vi "Get Measruement Informations.vi"(11 "Measurement properties":T1={"Measurement ID"=enum."1", "Description"="3 phase, 3 ADC, 1 PJVS", "Switching matrix M"=[], "Signal frequency  (Hz)"=50.0, "Signal amplitudes (V)"=[], "PRs"=1, "PRe"=50, "MRs"=0, "MRe"=0, "Set PJVS frequency (Hz)"=50.0, "PJVS reference voltages (1 period, V)"=[], "Requiested PJVS steps"=10} {"PJVS reference voltages (1 period, V)" format="%.9g"}) -> (3 "Measurement properties out":T1={"Measurement ID"=enum."1", "Description"="3 phase, 3 ADC, 1 PJVS", "Switching matrix M"=[], "Signal frequency  (Hz)"=50.0, "Signal amplitudes (V)"=[], "PRs"=1, "PRe"=50, "MRs"=0, "MRe"=0, "Set PJVS frequency (Hz)"=50.0, "PJVS reference voltages (1 period, V)"=[], "Requiested PJVS steps"=10} {"PJVS reference voltages (1 period, V)" format="%.9g"})   [LabVIEW 2020]
uses:
  Type definitions/Measuement properties.ctl
  Type definitions/Measurement ID.ctl
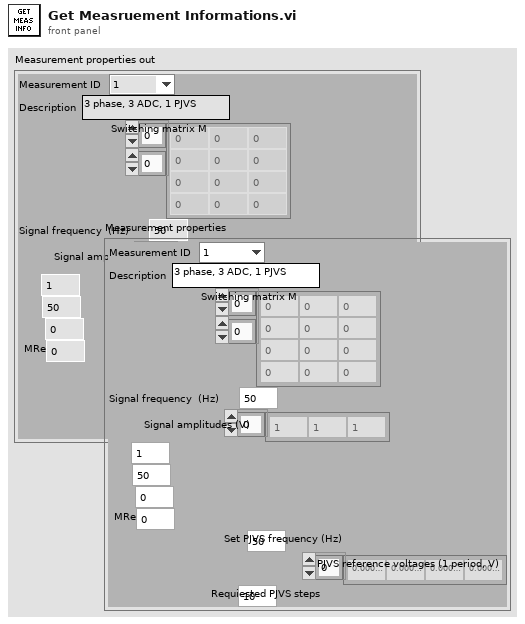
[diagram p1: front panel]
types:
  T1 = typedef "Measuement properties.ctl" = cluster{"Measurement ID":T2, "Description":string, "Switching matrix M":i32[][], "Signal frequency  (Hz)":dbl, "Signal amplitudes (V)":dbl[], "PRs":i32, "PRe":i32, "MRs":i32, "MRe":i32, "Set PJVS frequency (Hz)":dbl, "PJVS reference voltages (1 period, V)":dbl[], "Requiested PJVS steps":i32}
  T2 = typedef "Measurement ID.ctl" = enum16{"M", "1", "2", "3"}
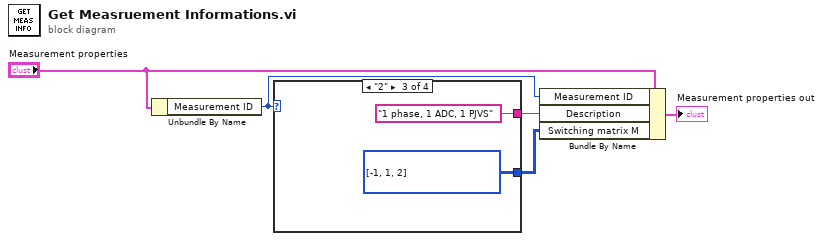
[diagram p0: block diagram]
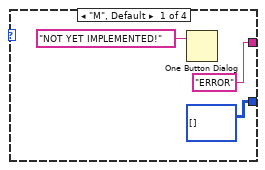
[diagram p2: hidden frame]
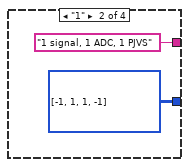
[diagram p3: hidden frame]
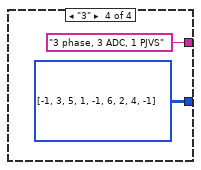
[diagram p4: hidden frame]
diagram:
  n1 = Unbundle By Name("Measurement properties") -> ("Measurement ID"=w1:T2)
  n2 = case shown="\"2\"" w1 {
    tunnel: ["ERROR" "1 signal, 1 ADC, 1 PJVS" "1 phase, 1 ADC, 1 PJVS" "3 phase, 3 ADC, 1 PJVS"] -> w4
    tunnel: [i32[][] [] ("M") i32[][] [[-1, 1], [1, -1]] ("M") i32[][] [[-1, 1, 2]] ("M") i32[][] [[-1, 3, 5], [1, -1, 6], [2, 4, -1]] ("M")] -> w3
    frame "M", Default {
      n3 = One Button Dialog(message="NOT YET IMPLEMENTED!") -> ()  [unwired: 1 in, 1 out]
    }
    frame "1" {
    }
    frame "2" {
    }
    frame "3" {
    }
  }
  n4 = Bundle By Name(cluster="Measurement properties", "Measurement ID"=w1, "Description"=w4, "Switching matrix M"=w3) -> (→"Measurement properties out":T1)
